vi "Actor Core.vi"(8 "error in":errorcluster, 11 "HIJ 4 Aligment Cams Launcher in":refnum<class "HIJ 3 Aligment Cams Launcher.lvclass">) -> (0 "error out":errorcluster, 3 "Actor out":refnum<class "Actor.lvclass">)   [LabVIEW 2014, in "HIJ 3 Alignment Cams App.lvlib" / "HIJ 3 Aligment Cams Launcher.lvclass"]
doc: "(<B>Filename</B>: Actor Framework.lvlib:Actor.lvclass:Actor Core.vi)\n\nReceives messages to the actor, reacts to them, and initiates any error handling that may shut the actor down.\n\nDescendant classes may override this VI to append parallel tasks for the actor to complete while it handles messages. Overrides use the Call Parent Method node."
uses:
  HIJ 3 Aligment Cams Launcher.lvclass
  <vilib>/ActorFramework/Actor/Actor.lvclass
  <vilib>/userdefined/High Color/IMAQdx.ctl
  HIJ 3 Alignment Cams App/HIJ 3 Alignment Cams App.lvclass
  HIJ Vision Launcher/HIJ Vision Launcher/HIJ Vision Launcher.lvclass/HIJ Vision Launcher.ctl
  Shared Code/Viewable Actor/ViewableActor/ViewableActor.lvclass/ViewableActor.ctl
  HIJ 3 Alignment Cams App/HIJ 3 Alignment Cams App.lvclass/HIJ 3 Alignment Cams App.ctl
  <vilib>/ActorFramework/Actor/Actor.lvclass/Actor.ctl
  <vilib>/ActorFramework/Message Enqueuer/Message Enqueuer.lvclass/Message Enqueuer.ctl
  HIJ 3 Aligment Cams Launcher Messages/Set Sart Cameras Msg/Set Sart Cameras Msg.lvclass/Set Sart Cameras Msg.ctl
  HIJ Vision Launcher/HIJ Vision Launcher/Read HIJ Vision Camera App.vi
  HIJ Vision Launcher/HIJ Vision Launcher/Read Cmd Parameters.vi
  Shared Code/Viewable Actor/ViewableActor/Read Config URL.vi
  HIJ 3 Alignment Cams App/Write Start Camera 3.vi
  HIJ 3 Alignment Cams App/Write Start Camera 2.vi
  HIJ Vision Launcher/HIJ Vision Launcher/Write HIJ Vision Camera App.vi
  <vilib>/ActorFramework/Message Enqueuer/Init from Existing Queue.vi
  <vilib>/ActorFramework/Message Enqueuer/Enqueue.vi
  <vilib>/Utility/config.llb/Read Key (String).vi
  <vilib>/Utility/config.llb/Write Key (String).vi
  <vilib>/ActorFramework/Message Priority Queue/Priority Enqueue.vi
  Shared Code/Viewable Actor/ViewableActor/ViewableActor.lvclass
  <vilib>/ActorFramework/Message Enqueuer/Message Enqueuer.lvclass
  HIJ 3 Aligment Cams Launcher Messages/Set Sart Cameras Msg/Set Sart Cameras Msg.lvclass
  <vilib>/ActorFramework/Stop Msg/Stop Msg.lvclass
  HIJ Vision Launcher/HIJ Vision Launcher/HIJ Vision Launcher.lvclass
  <vilib>/Utility/config.llb/NI_LVConfig.lvlib
panel:
  in  "Camera 2":T1="dummy"
  in  "Camera 3":T1="dummy"
  in  "RUN_STOP":bool
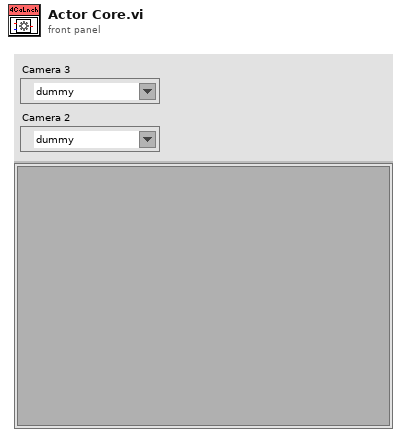
[diagram p1: front panel]
types:
  T1 = typedef "IMAQdx.ctl" = refnum<k21>
  T2 = typedef "NI_LVConfig.lvlib/Config Data RefNum.ctl" = refnum<k1>
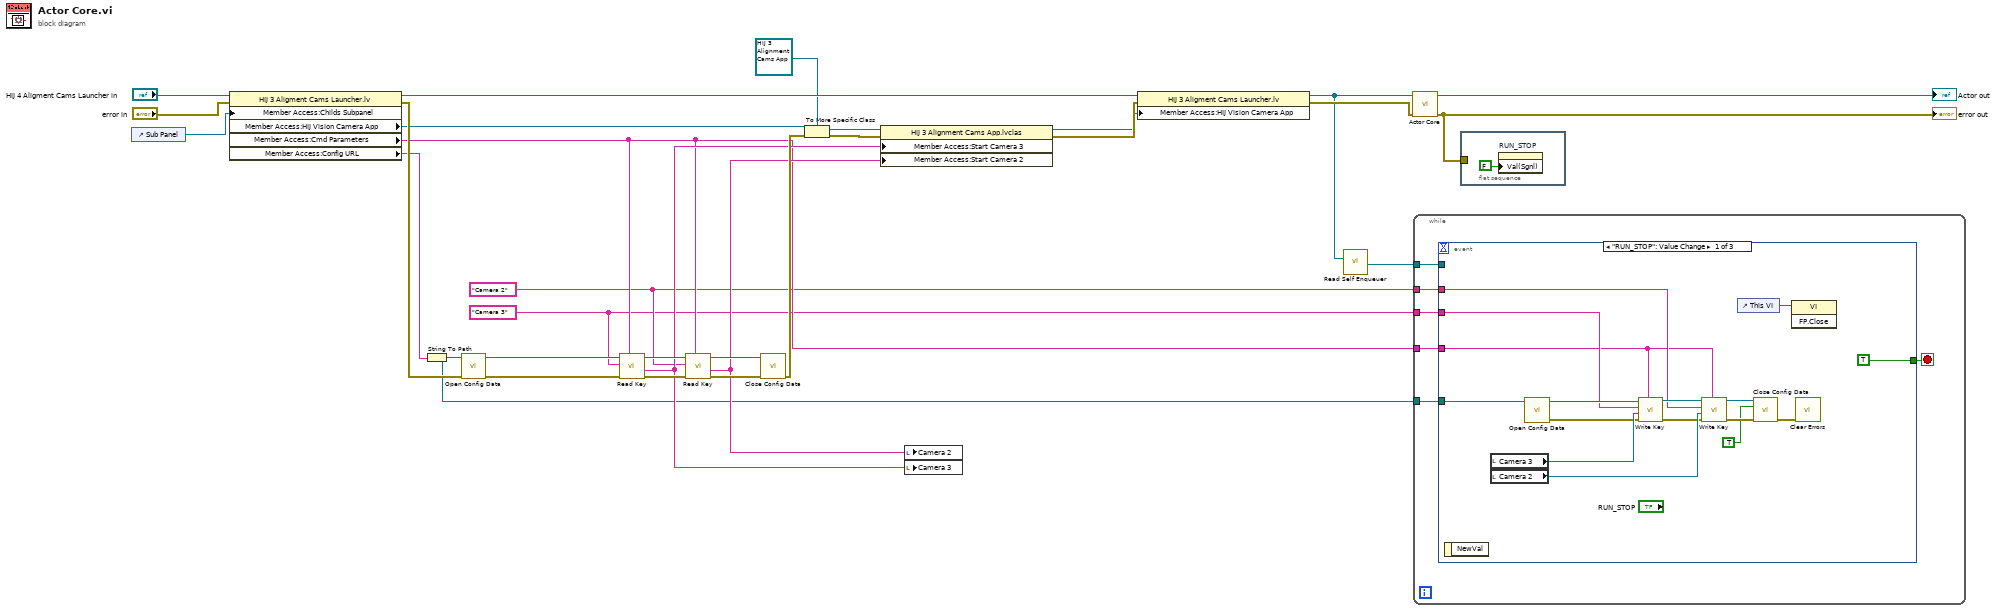
[diagram p0: block diagram]
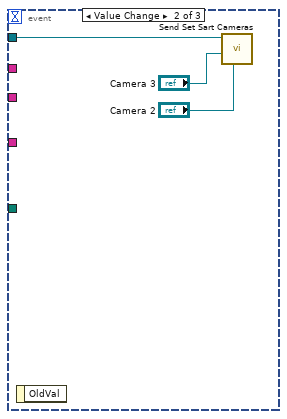
[diagram p2: hidden frame]
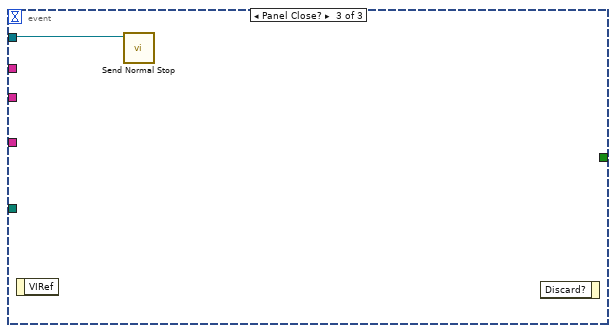
[diagram p3: hidden frame]
diagram:
  w9 = "Camera 2" ("key")
  w8 = "Camera 3" ("key")
  n1 = control-ref of="Sub Panel"() -> (w25:refnum<vi>)
  n2 = property class="HIJ 3 Aligment Cams Launcher.lv"(reference="HIJ 4 Aligment Cams Launcher in", error in="error in", "Member Access:Childs Subpanel"=w25) -> (reference out=w26:refnum<class "HIJ 3 Aligment Cams Launcher.lvclass">, error out=w29:errorcluster, "Member Access:HIJ Vision Camera App"=w4:refnum<class "ViewableActor.lvclass">, "Member Access:Cmd Parameters"=w10:string, "Member Access:Config URL"=w24:string)
  n3 = String To Path(string=w24) -> (path=w15:path)
  n4 = call <vilib>:"Open Config Data.vi"("error in (no error)"=w29, "configuration file path"=w15) -> ("error out"=w23:errorcluster, "refnum"=w22:T2)  [unwired: 7 in, 1 out]
  n5 = call-poly <vilib>:"Read Key.vi"("section"=w10, "error in (no error)"=w23, "key"=w8, "refnum"=w22) -> ("error out"=w20:errorcluster, "value"=w17:string, "refnum out"=w21:T2)  [unwired: 4 in, 1 out]
  n6 = call-poly <vilib>:"Read Key.vi"("section"=w10, "error in (no error)"=w20, "key"=w9, "refnum"=w21) -> ("error out"=w18:errorcluster, "value"=w16:string, "refnum out"=w19:T2)  [unwired: 4 in, 1 out]
  n7 = call <vilib>:"Close Config Data.vi"("error in (no error)"=w18, "refnum"=w19) -> ("error out"=w30:errorcluster)  [unwired: 8 in, 1 out]
  n8 = To More Specific Class(target class=refnum<class "HIJ 3 Alignment Cams App.lvclass"> refnum ("HIJ 4 Alignment Cams App.lvlib:HIJ 4 Alignment Cams App.lvclass"), reference=w4, error in=w30) -> (specific class reference=w1:refnum<class "HIJ 3 Alignment Cams App.lvclass">, error out=w3:errorcluster)
  n9 = property class="HIJ 3 Alignment Cams App.lvclas"(reference=w1, error in=w3, "Member Access:Start Camera 3"=w17, "Member Access:Start Camera 2"=w16) -> (reference out=w2:refnum<class "HIJ 3 Alignment Cams App.lvclass">, error out=w13:errorcluster)
  n10 = local write "Camera 2"(w16) -> ()
  n11 = local write "Camera 3"(w17) -> ()
  n12 = property class="HIJ 3 Aligment Cams Launcher.lv"(reference=w26, error in=w13, "Member Access:HIJ Vision Camera App"=w2) -> (reference out=w11:refnum<class "HIJ 3 Aligment Cams Launcher.lvclass">, error out=w12:errorcluster)
  n13 = call <vilib>:"Read Self Enqueuer.vi"("Actor"=w11) -> ("Self Enqueuer"=w7:refnum<class "Message Enqueuer.lvclass">)  [unwired: 10 in]
  n14 = call-parent "Actor Core.vi"("error in"=w12, "HIJ Vision Launcher in"=w11) -> ("error out"=w6:errorcluster, "Actor out"=→"Actor out":refnum<class "Actor.lvclass">)  [unwired: 8 in]
  "error out" <- w6
  n15 = while {
    tunnel: w10 -> [w35]
    tunnel: w15 -> [w34]
    tunnel: w8 -> [w33]
    tunnel: w9 -> [w32]
    tunnel: w7 -> [w31]
    stop <- w36 stop-if-true
    n16 = event shown="[0] \"RUN_STOP\": Value Change" {
      selector: _ -> [_ _ _]
      dyn-events: _ -> [_ _ _]
      timeout: _ -> [_ _ _]
      tunnel: [TRUE _ _] -> w36
      tunnel: w35 -> [w39 _ _]
      tunnel: w34 -> [w43 _ _]
      tunnel: w33 -> [w41 _ _]
      tunnel: w32 -> [w40 _ _]
      tunnel: w31 -> [_ w55 w56]
      event "RUN_STOP": Value Change {
        n17 = event-data() -> ()  [unwired: 1 in, 1 out]
        n18 = local read "Camera 3"() -> (w50:T1)
        n19 = local read "Camera 2"() -> (w51:T1)
        n20 = call <vilib>:"Open Config Data.vi"("configuration file path"=w43) -> ("error out"=w37:errorcluster, "refnum"=w42:T2)  [unwired: 8 in, 1 out]
        n21 = call-poly <vilib>:"Write Key.vi"("section"=w39, "error in (no error)"=w37, "value"=w50, "key"=w41, "refnum"=w42) -> ("error out"=w48:errorcluster, "refnum out"=w49:T2)  [unwired: 4 in, 1 out]
        n22 = call-poly <vilib>:"Write Key.vi"("section"=w39, "error in (no error)"=w48, "value"=w51, "key"=w40, "refnum"=w49) -> ("error out"=w47:errorcluster, "refnum out"=w46:T2)  [unwired: 4 in, 1 out]
        n23 = control-ref of="This VI"() -> (w38:refnum<vi>)
        n24 = call <vilib>:"Close Config Data.vi"("error in (no error)"=w47, "write file if changed (T)"=TRUE, "refnum"=w46) -> ("error out"=w44:errorcluster)  [unwired: 7 in, 1 out]
        n25 = invoke class="VI" method="FP.Close"(reference=w38) -> ()  [unwired: 2 in, 3 out]
        n26 = call <vilib>:"Clear Errors.vi"("error in (no error)"=w44) -> ()  [unwired: 5 in, 2 out]
      }
      event Value Change {
        n27 = event-data() -> ()  [unwired: 1 in, 1 out]
        n28 = call "Send Set Sart Cameras.vi"("Camera 2"="Camera 2", "Camera 3"="Camera 3", "Message Enqueuer"=w55) -> ()  [unwired: 7 in, 2 out]
      }
      event Panel Close? {
        n29 = event-data() -> ()  [unwired: 1 in, 1 out]
        n30 = call <vilib>:"Send Normal Stop.vi"("Message Enqueuer"=w56) -> ()  [unwired: 10 in, 1 out]
        n31 = event-data() -> ()  [unwired: 2 in, 1 out]
      }
    }
  }
  n32 = flat-sequence {
    tunnel: w6 -> [_]
    frame #0 {
      n33 = property on="RUN_STOP" class="Bool (strict)"("Val(Sgnl)"=FALSE ("Value (Signaling)")) -> ()  [unwired: 2 in, 2 out]
    }
  }
